vi "WPI_AnalogChannelERRChannelAllocated.vi"(8 "error in (no error)":errorcluster, 10 "AI Channel":T2=enum."Invalid", 11 "AO Channel":T1=enum."Invalid") -> (0 "ERRChannelAllocated":errorcluster)   [LabVIEW 2017]
doc: "This software is licensed. Open the labview\\readme\\WPI Robotics Library Open Source License.txt file for more information."
uses:
  <vilib>/Rock Robotics/SystemInterfaces/AI/FPGA_AIChannel.ctl
  <vilib>/Rock Robotics/WPI/AnalogOutput/WPI_AnalogOutputChannel.ctl
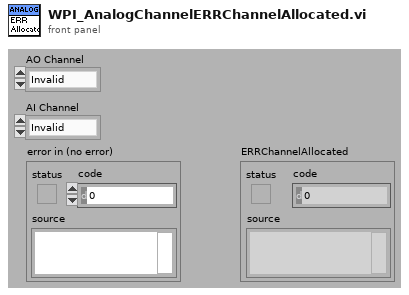
[diagram p1: front panel]
types:
  T1 = typedef "WPI_AnalogOutputChannel.ctl" = enum8{"AO MXP 0", "AO MXP 1", "Invalid"}
  T2 = typedef "FPGA_AIChannel.ctl" = enum8{"AI 0", "AI 1", "AI 2", "AI 3", "AI MXP 0", "AI MXP 1", "AI MXP 2", "AI MXP 3", "Invalid"}
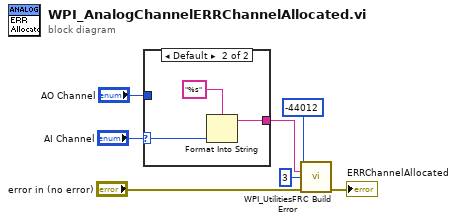
[diagram p0: block diagram]
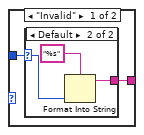
[diagram p2: hidden frame]
diagram:
  n1 = case shown="Default" "AI Channel" {
    selector: "AI Channel" -> [_ w15]
    tunnel: [w9 w14] -> w2
    tunnel: "AO Channel" -> [w8 _]
    frame "Invalid" {
      n2 = case shown="Default" w8 {
        selector: w8 -> [_ w10]
        tunnel: [_ w11] -> w9
        frame "Invalid" {
        }
        frame Default {
          n3 = Format Into String(format string="%s", w10) -> (resulting string=w11:string)  [unwired: 2 in, 1 out]
        }
      }
    }
    frame Default {
      n4 = Format Into String(format string="%s", w15) -> (resulting string=w14:string)  [unwired: 2 in, 1 out]
    }
  }
  n5 = call <vilib>:"WPI_UtilitiesFRC Build Error.vi"("error code"=-44012 ("code"), "extra error text"=w2, "chain levels to remove (1)"=3, "error in (no error)"="error in (no error)") -> ("error out"=→"ERRChannelAllocated":errorcluster)  [unwired: 1 in, 10 out]
